vi "Pure Pursuit_New (Sub VI).vi"(0 "x_lat_path":dbl[](array[numeric]), 2 "L":dbl format="%#_13g", 5 "y_long_path":dbl[](array[numeric]), 7 "X_Current":dbl format="%#_13g", 9 "Y_Current":dbl format="%#_13g", 11 "Heading_Current":dbl format="%#_13g", 12 "#pnt":i32, 13 "WP no_pre":i32, 14 "LAD":dbl format="%#_13g") -> (4 "Steer_CMD(Deg)":dbl, 8 "숫자형":dbl, 10 "숫자형 2":dbl, 15 "Index(near vehicle)":i32)   [LabVIEW 2024]
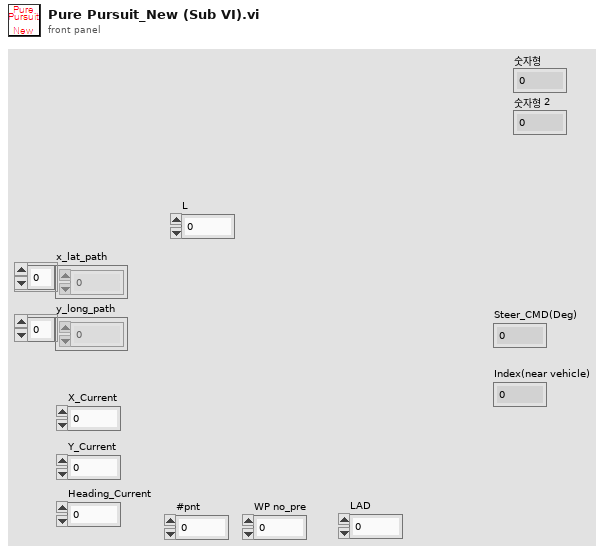
[diagram p1: front panel]
types:
  T1 = cluster{"Dist. WP":dbl, "Index":i32, "Heading_lane":dbl, "Dist. lane":dbl}
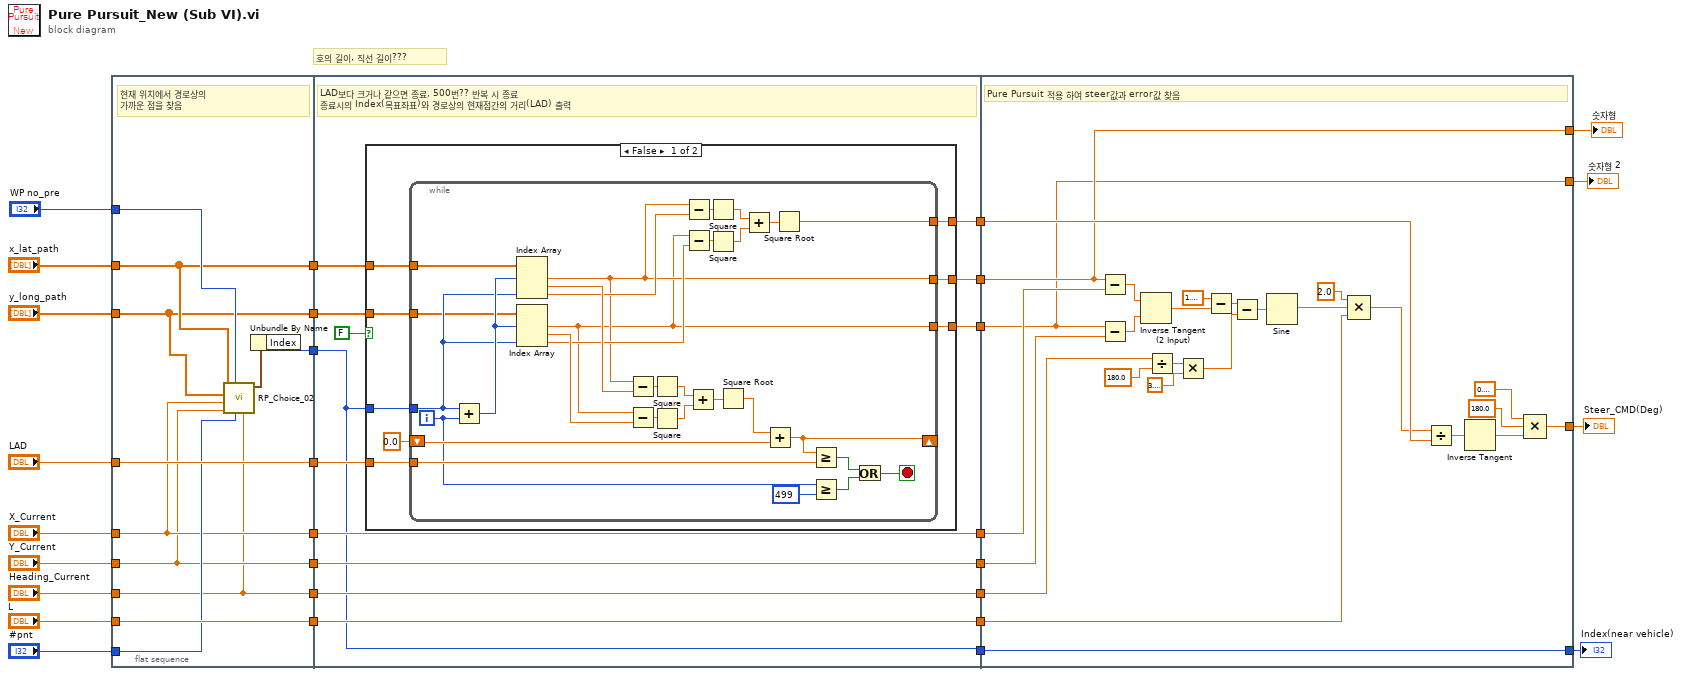
[diagram p0: block diagram]
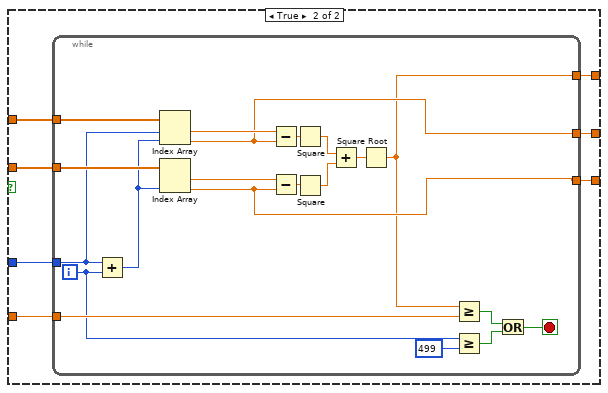
[diagram p2: hidden frame]
diagram:
  # "호의 길이, 직선 길이???"
  n1 = flat-sequence {
    tunnel: "x_lat_path" -> [w36]
    tunnel: [w36] -> w29
    tunnel: "y_long_path" -> [w35]
    tunnel: [w35] -> w27
    tunnel: "LAD" -> [w40]
    tunnel: [w40] -> w24
    tunnel: "X_Current" -> [w34]
    tunnel: "Y_Current" -> [w33]
    tunnel: [w34] -> w20
    tunnel: [w33] -> w19
    tunnel: "Heading_Current" -> [w30]
    tunnel: [w30] -> w15
    tunnel: "L" -> [w39]
    tunnel: [w39] -> w11
    tunnel: "WP no_pre" -> [w38]
    tunnel: "#pnt" -> [w37]
    tunnel: [w31] -> w5
    tunnel: w29 -> [w52]
    tunnel: w27 -> [w51]
    tunnel: w24 -> [w50]
    tunnel: [w49] -> w23
    tunnel: [w48] -> w22
    tunnel: [w47] -> w21
    tunnel: w20 -> [w46]
    tunnel: w19 -> [w45]
    tunnel: [w46] -> w18
    tunnel: [w45] -> w17
    tunnel: w15 -> [w44]
    tunnel: [w44] -> w14
    tunnel: [w43] -> w13
    tunnel: w11 -> [w43]
    tunnel: [w41] -> w10
    tunnel: w5 -> [w41]
    tunnel: w23 -> [w137]
    tunnel: w22 -> [w119]
    tunnel: w21 -> [w118]
    tunnel: w18 -> [w131]
    tunnel: w17 -> [w130]
    tunnel: w14 -> [w125]
    tunnel: w13 -> [w121]
    tunnel: w10 -> [w143]
    tunnel: [w143] -> w9
    tunnel: [w139] -> w8
    tunnel: [w119] -> w4
    tunnel: [w118] -> w3
    frame #0 {
      # "현재 위치에서 경로상의\n가까운 점을 찾음"
      n2 = call "RP_Choice_02.vi"("Heading_c"=w30, "# of pnt"=w37, "WP no_pre"=w38, "y_long_c"=w33, "x_lat_c"=w34, "y_long_arr"=w35, "x_lat_arr"=w36) -> ("RP1"=w32:T1)  [unwired: 1 in, 3 out]
      n3 = Unbundle By Name(w32) -> ("Index"=w31:i32)
    }
    frame #1 {
      # "LAD보다 크거나 같으면 종료, 500번?? 반복 시 종료\n종료시의 Index(목표좌표)와 경로상의 현재점간의 거리(LAD) 출력"
      n4 = case shown="False" FALSE {
        tunnel: w41 -> [w57 w97]
        tunnel: w52 -> [w59 w96]
        tunnel: w51 -> [w58 w95]
        tunnel: w50 -> [w53 w94]
        tunnel: [w54 w93] -> w49
        tunnel: [w55 w92] -> w48
        tunnel: [w56 w91] -> w47
        frame False {
          n5 = while {
            tunnel: w57 -> [w89]
            tunnel: w59 -> [w83]
            tunnel: w58 -> [w82]
            tunnel: w53 -> [w77]
            shift-right: [w76] -> _
            shift-left: 0.0 -> [w78]
            tunnel: [w63] -> w54
            tunnel: [w62] -> w55
            tunnel: [w61] -> w56
            i -> [w72]
            stop <- w73 stop-if-true
            n6 = Add(x=w89, y=w72) -> (x+y=w90:i32)
            n7 = Index Array(array=w83, index #1=w90, index #3=w89) -> (element #1=w62:dbl, element #2=w81:dbl, element #3=w65:dbl)  [unwired: 1 in]
            n8 = Index Array(array=w82, index #1=w90, index #3=w89) -> (element #1=w61:dbl, element #2=w80:dbl, element #3=w64:dbl)  [unwired: 1 in]
            n9 = Subtract(x=w62, y=w81) -> (x-y=w87:dbl)
            n10 = Subtract(x=w61, y=w80) -> (x-y=w88:dbl)
            n11 = Square(x=w87) -> (x^2=w86:dbl)
            n12 = Square(x=w88) -> (x^2=w85:dbl)
            n13 = Subtract(x=w62, y=w65) -> (x-y=w67:dbl)
            n14 = Subtract(x=w61, y=w64) -> (x-y=w66:dbl)
            n15 = Add(x=w86, y=w85) -> (x+y=w84:dbl)
            n16 = Square(x=w67) -> (x^2=w68:dbl)
            n17 = Square(x=w66) -> (x^2=w69:dbl)
            n18 = Square Root(x=w84) -> (sqrt(x)=w79:dbl)
            n19 = Add(x=w68, y=w69) -> (x+y=w70:dbl)
            n20 = Add(x=w79, y=w78) -> (x+y=w76:dbl)
            n21 = Square Root(x=w70) -> (sqrt(x)=w63:dbl)
            n22 = Greater Or Equal?(x=w76, y=w77) -> (x >= y?=w75:bool)
            n23 = Greater Or Equal?(x=w72, y=499) -> (x >= y?=w74:bool)
            n24 = Or(x=w75, y=w74) -> (x .or. y?=w73:bool)
          }
        }
        frame True {
          n25 = while {
            tunnel: w97 -> [w103]
            tunnel: w96 -> [w112]
            tunnel: w95 -> [w111]
            tunnel: w94 -> [w110]
            tunnel: [w98] -> w93
            tunnel: [w100] -> w92
            tunnel: [w99] -> w91
            i -> [w106]
            stop <- w107 stop-if-true
            n26 = Add(x=w103, y=w106) -> (x+y=w104:i32)
            n27 = Index Array(array=w112, index #1=w103, index #2=w104) -> (element #1=w102:dbl, element #2=w100:dbl)
            n28 = Index Array(array=w111, index #2=w104) -> (element #1=w101:dbl, element #2=w99:dbl)  [unwired: 1 in]
            n29 = Subtract(x=w102, y=w100) -> (x-y=w116:dbl)
            n30 = Subtract(x=w101, y=w99) -> (x-y=w117:dbl)
            n31 = Square(x=w116) -> (x^2=w115:dbl)
            n32 = Square(x=w117) -> (x^2=w114:dbl)
            n33 = Add(x=w115, y=w114) -> (x+y=w113:dbl)
            n34 = Square Root(x=w113) -> (sqrt(x)=w98:dbl)
            n35 = Greater Or Equal?(x=w98, y=w110) -> (x >= y?=w109:bool)
            n36 = Greater Or Equal?(x=w106, y=499) -> (x >= y?=w108:bool)
            n37 = Or(x=w109, y=w108) -> (x .or. y?=w107:bool)
          }
        }
      }
    }
    frame #2 {
      # "Pure Pursuit 적용 하여 steer값과 error값 찾음"
      n38 = Subtract(x=w119, y=w131) -> (x-y=w136:dbl)
      n39 = Subtract(x=w118, y=w130) -> (x-y=w135:dbl)
      n40 = Inverse Tangent (2 Input)(1:w135, 2:w136) -> (0:w134:dbl)
      n41 = Divide(x=w125, y=180.0) -> (x/y=w129:dbl)
      n42 = Multiply(x=w129, y=3.141592653589793) -> (x*y=w127:dbl)
      n43 = Subtract(x=1.5707963267948966, y=w134) -> (x-y=w133:dbl)
      n44 = Subtract(x=w133, y=w127) -> (x-y=w124:dbl)
      n45 = Sine(x=w124) -> (sin(x)=w122:dbl)
      n46 = Compound Arithmetic op=MULTIPLY(2.0, w122, w121) -> (w120:dbl)
      n47 = Divide(x=w120, y=w137) -> (x/y=w138:dbl)
      n48 = Inverse Tangent(1:w138) -> (0:w140:dbl)
      n49 = Compound Arithmetic op=MULTIPLY(0.3183098861837907, 180.0, w140) -> (w139:dbl)
    }
  }
  "Steer_CMD(Deg)" <- w8
  "Index(near vehicle)" <- w9
  "숫자형" <- w4
  "숫자형 2" <- w3
